vi "Step.vi"(8 "error in":errorcluster, 11 "GoL in":refnum<class "GoL.lvclass">) -> (0 "error out":errorcluster, 2 "Grid":u8[][](array[numeric]), 3 "GoL out":refnum<class "GoL.lvclass">)   [LabVIEW 2026, in "GoL.lvlib" / "GoL.lvclass"]
uses:
  GoL.lvclass
  GoL.lvclass/GoL.ctl
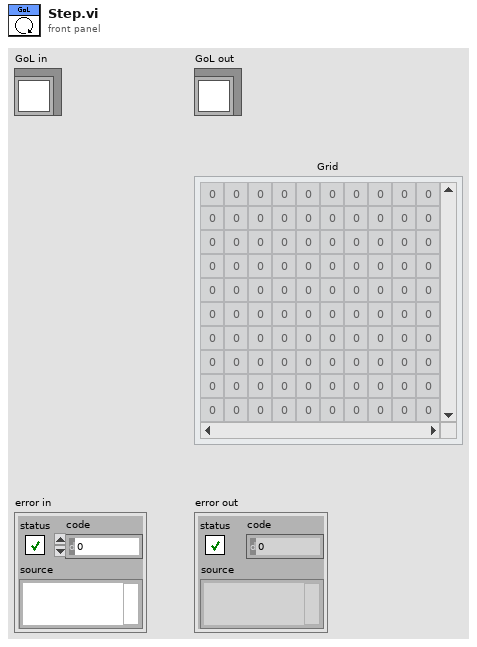
[diagram p1: front panel]
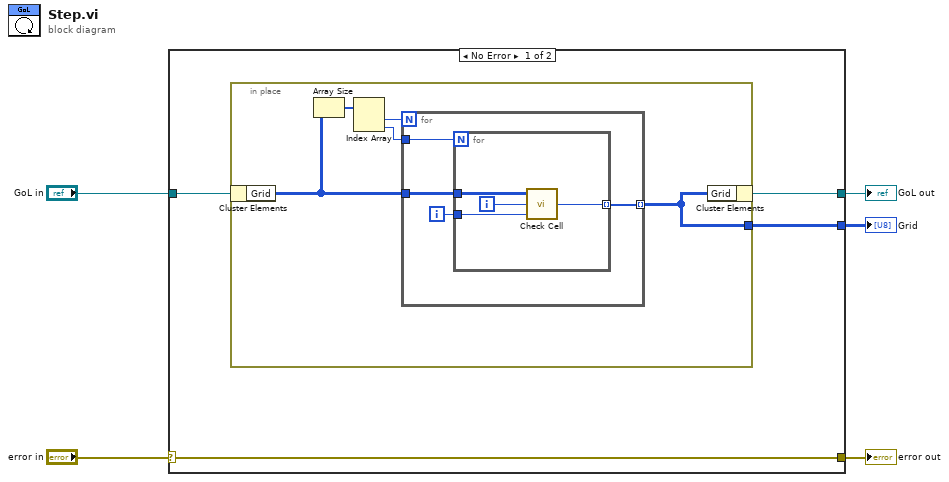
[diagram p0: block diagram]
diagram:
  n1 = case shown="No Error" "error in" {
    selector: "error in" -> [w9 w24]
    tunnel: [w9 w24] -> w4
    tunnel: [w7 w23] -> w2
    tunnel: "GoL in" -> [w8 w23]
    tunnel: [w6 _] -> w1
    frame No Error {
      n2 = in-place {
        in-place-border: [w10] -> w6
        n3 = in-place-cluster #1(w8) -> ("Grid"=w13:u8[][])
        n4 = Array Size(array=w13) -> (size(s)=w14:i32[])
        n5 = Index Array(array=w14) -> (element #1=w12:i32, element #2=w11:i32)  [unwired: 2 in]
        n6 = for {
          N: w12 -> [_]
          tunnel: w13 -> [w18]
          tunnel: w11 -> [w17]
          tunnel: [w15] -> w10 mode=indexing
          i -> [w16]
          n7 = for {
            N: w17 -> [_]
            tunnel: w18 -> [w22]
            tunnel: w16 -> [w20]
            tunnel: [w19] -> w15 mode=indexing
            i -> [w21]
            n8 = call "Check Cell.vi"("y"=w20, "x"=w21, "Grid"=w22) -> ("Cell"=w19:u8)
          }
        }
        n9 = in-place-cluster #1("Grid"=w10) -> (w7:refnum<class "GoL.lvclass">)
      }
    }
    frame Error {
    }
  }
  "error out" <- w4
  "GoL out" <- w2
  "Grid" <- w1
